vi "sinewave.vi"() -> ()   [LabVIEW 2019]
uses:
  <vilib>/DAQmx/write.llb/DAQmx Write (Analog 1D DBL 1Chan NSamp).vi
  <vilib>/DAQmx/write.llb/DAQmx Write (Analog DBL 1Chan 1Samp).vi
  <vilib>/DAQmx/create/channels.llb/DAQmx Create Channel (AO-Voltage-Basic).vi
  <vilib>/DAQmx/create/channels.llb/DAQmx Create Channel (CO-Pulse Generation-Ticks).vi
  <vilib>/DAQmx/configure/timing.llb/DAQmx Timing (Sample Clock).vi
  <vilib>/DAQmx/miscellaneous.llb/DAQmx Fill In Error Info.vi
  <vilib>/DAQmx/configure/timing.llb/DAQmx Timing (Implicit).vi
  <resource>/objmgr/daqmx.rc
panel:
  in  "stop":bool
  out "Array":dbl[](array[numeric])
  in  "frequency":dbl=100.0 format="%#_13g"
  in  "amplitude":dbl=5.0 format="%.3f"
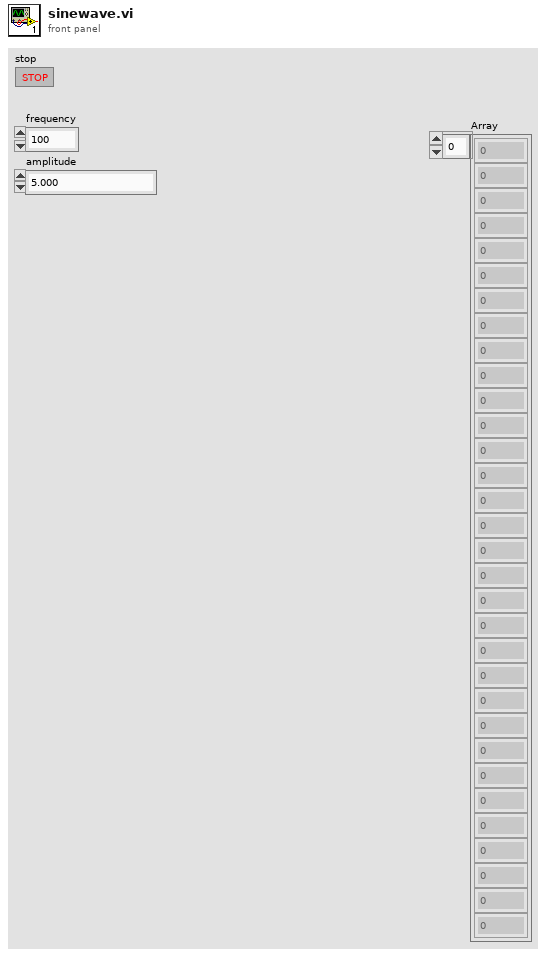
[diagram p1: front panel]
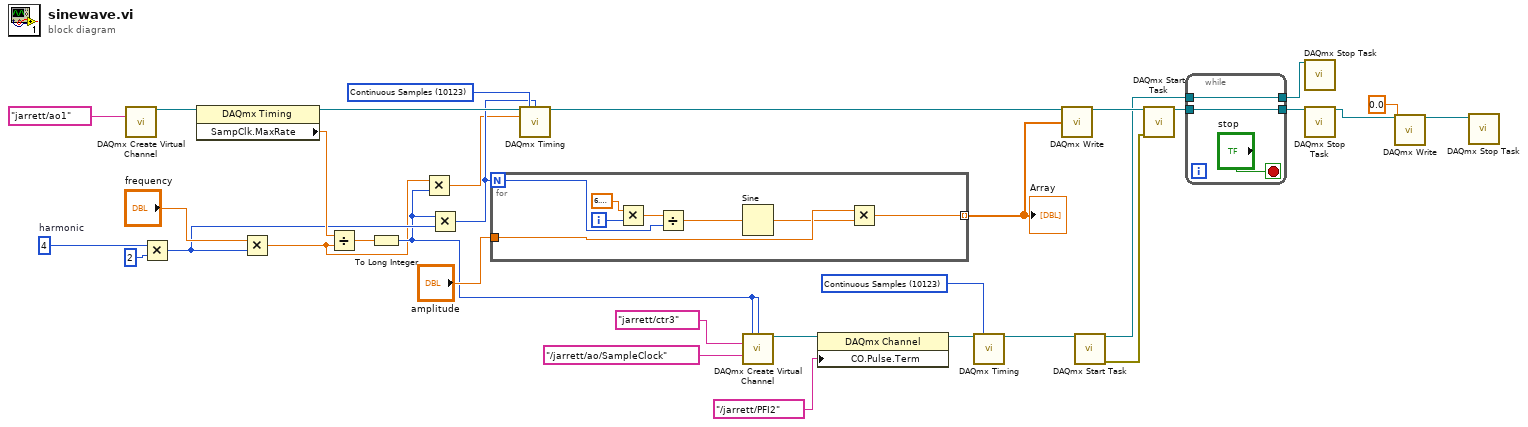
[diagram p0: block diagram]
diagram:
  w13 = 10123 items=["Finite Samples"=10178, "Continuous Samples"=10123, "Hardware Timed Single Point"=12522] ("sample mode")
  w26 = 10123 items=["Finite Samples"=10178, "Continuous Samples"=10123, "Hardware Timed Single Point"=12522] ("sample mode")
  w11 = 4  # harmonic
  n1 = call-poly <vilib>:"DAQmx Create Virtual Channel.vi"("physical channels"=tag "jarrett/ao1") -> ("task out"=w27:refnum<k21>)  [unwired: 13 in, 1 out]
  n2 = Multiply(x=w11, y=2) -> (x*y=w8:i32)
  n3 = property class="DAQmx Timing"(reference=w27) -> (reference out=w12:refnum<k21>, "SampClk.MaxRate"=w10:dbl)  [unwired: 1 in, 1 out]
  n4 = Multiply(x="frequency", y=w8) -> (x*y=w5:dbl)
  n5 = Divide(x=w10, y=w5) -> (x/y=w9:dbl)
  n6 = To Long Integer(number=w9) -> (32bit integer=w6:i32)
  n7 = Multiply(x=w5, y=w6) -> (x*y=w4:dbl)
  n8 = Multiply(x=w6, y=w8) -> (x*y=w7:i32)
  n9 = for {
    N: w7 -> [w36]
    tunnel: "amplitude" -> [w41]
    tunnel: [w34] -> w24 mode=indexing
    i -> [w39]
    n10 = Multiply(x=6.283185307179586, y=w39) -> (x*y=w37:dbl)
    n11 = Divide(x=w37, y=w36) -> (x/y=w35:dbl)
    n12 = Sine(x=w35) -> (sin(x)=w40:dbl)
    n13 = Multiply(x=w41, y=w40) -> (x*y=w34:dbl)
  }
  "Array" <- w24
  n14 = call-poly <vilib>:"DAQmx Timing.vi"("task/channels in"=w12, "sample mode"=w26, "samples per channel"=w7, "rate"=w4) -> ("task out"=w25:refnum<k21>)  [unwired: 10 in, 1 out]
  n15 = call-poly <vilib>:"DAQmx Create Virtual Channel.vi"("high ticks"=w6, "low ticks"=w6, "counter"=tag "jarrett/ctr3", "source of ticks"=tag "/jarrett/ao/SampleClock") -> ("task out"=w23:refnum<k21>)  [unwired: 10 in, 1 out]
  n16 = property class="DAQmx Channel"(reference=w23, "CO.Pulse.Term"=tag "/jarrett/PFI2") -> (reference out=w15:refnum<k21>)  [unwired: 1 in, 1 out]
  n17 = call-poly <vilib>:"DAQmx Timing.vi"("task/channels in"=w15, "sample mode"=w13) -> ("task out"=w14:refnum<k21>)  [unwired: 12 in, 1 out]
  n18 = call-poly <vilib>:"DAQmx Write.vi"("task/channels in"=w25, "data"=w24) -> ("task out"=w21:refnum<k21>)  [unwired: 11 in, 2 out]
  n19 = call <vilib>:"DAQmx Start Task.vi"("task/channels in"=w14) -> ("task out"=w17:refnum<k21>, "error out"=w22:errorcluster)  [unwired: 13 in]
  n20 = call <vilib>:"DAQmx Start Task.vi"("task/channels in"=w21, "error in"=w22) -> ("task out"=w19:refnum<k21>)  [unwired: 12 in, 1 out]
  n21 = while {
    tunnel: [w43] -> w20
    tunnel: w19 -> [w43]
    tunnel: [w42] -> w18
    tunnel: w17 -> [w42]
    stop <- "stop" stop-if-true
  }
  n22 = call <vilib>:"DAQmx Stop Task.vi"("task/channels in"=w18) -> ()  [unwired: 13 in, 2 out]
  n23 = call <vilib>:"DAQmx Stop Task.vi"("task/channels in"=w20) -> ("task out"=w3:refnum<k21>)  [unwired: 13 in, 1 out]
  n24 = call-poly <vilib>:"DAQmx Write.vi"("task/channels in"=w3, "data"=0.0) -> ("task out"=w1:refnum<k21>)  [unwired: 11 in, 2 out]
  n25 = call <vilib>:"DAQmx Stop Task.vi"("task/channels in"=w1) -> ()  [unwired: 13 in, 2 out]
